vi "Write all.vi"(7 "Zentrum":dbl[](array[numeric]), 8 "error in (no error)":errorcluster, 9 "Radius":dbl, 10 "Sektor":T1(ring), 11 "Kreisquadrant in":refnum<class "Kreisquadrant.lvclass">) -> (0 "error out":errorcluster, 3 "Kreisquadrant out":refnum<class "Kreisquadrant.lvclass">)   [LabVIEW 2019, in "Kreisquadrant.lvclass"]
uses:
  Kreisquadrant.lvclass
  Kreisquadrant.lvclass/Kreisquadrant.ctl
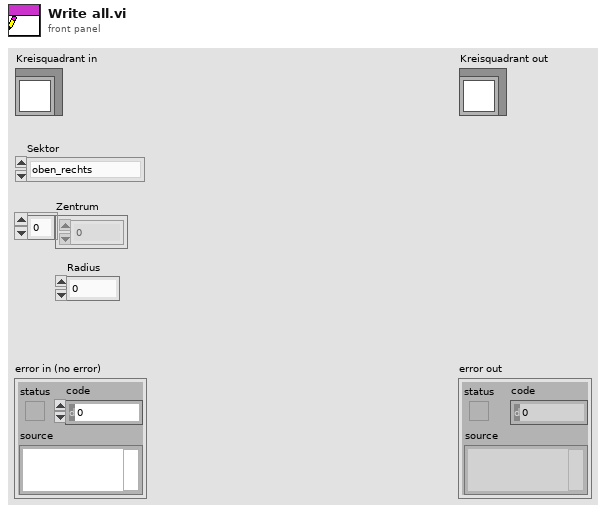
[diagram p1: front panel]
types:
  T1 = enum16{"oben_rechts", "oben_links", "unten_links", "unten_rechts"}
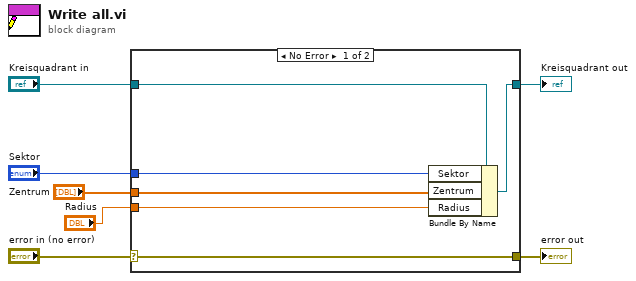
[diagram p0: block diagram]
diagram:
  n1 = case shown="No Error" "error in (no error)" {
    selector: "error in (no error)" -> [w13 w14]
    tunnel: [w13 w14] -> w6
    tunnel: [w11 w15] -> w4
    tunnel: "Kreisquadrant in" -> [w12 w15]
    tunnel: "Sektor" -> [w10 _]
    tunnel: "Radius" -> [w9 _]
    tunnel: "Zentrum" -> [w8 _]
    frame No Error {
      n2 = Bundle By Name(cluster=w12, "Sektor"=w10, "Zentrum"=w8, "Radius"=w9) -> (w11:refnum<class "Kreisquadrant.lvclass">)
    }
    frame Error {
    }
  }
  "error out" <- w6
  "Kreisquadrant out" <- w4
